vi "Read Child Items.vi"(8 "error in":errorcluster, 11 "Item in":refnum<class "Item.lvclass">) -> (0 "error out":errorcluster, 2 "Child Items":cluster{"Type":T1, "Value":variant}[](array[cluster]), 3 "Item out":refnum<class "Item.lvclass">)   [LabVIEW 2024, in "Config File Parser.lvlib" / "Item.lvclass"]
uses:
  Item.lvclass
  Item Type.ctl
  Item.lvclass/Item.ctl
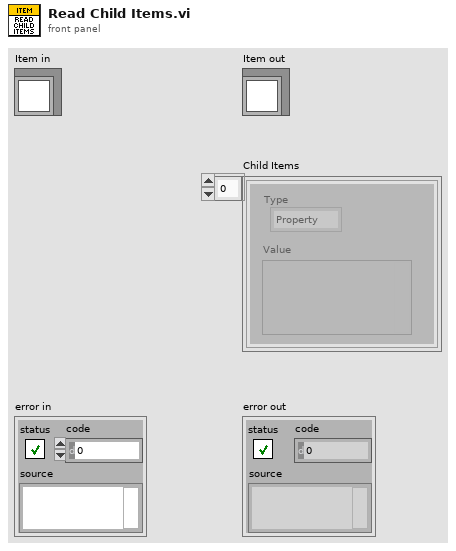
[diagram p1: front panel]
types:
  T1 = typedef "Config File Parser.lvlib/Item.lvclass/Item Type.ctl" = enum16{"Property", "Channel", "Section"}
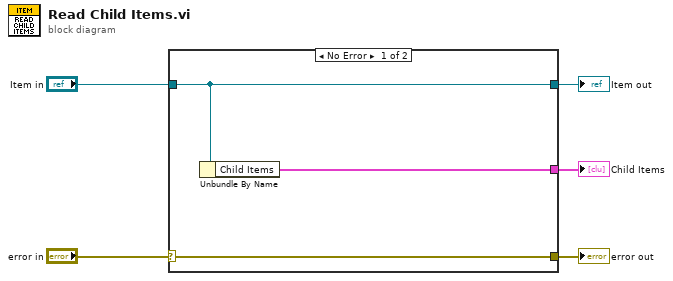
[diagram p0: block diagram]
diagram:
  n1 = case shown="No Error" "error in" {
    selector: "error in" -> [w8 w10]
    tunnel: [w8 w10] -> w4
    tunnel: [w7 w9] -> w2
    tunnel: "Item in" -> [w7 w9]
    tunnel: [w6 _] -> w1
    frame No Error {
      n2 = Unbundle By Name(w7) -> ("Child Items"=w6:cluster{"Type":T1, "Value":variant}[])
    }
    frame Error {
    }
  }
  "error out" <- w4
  "Item out" <- w2
  "Child Items" <- w1
